vi "Votlage - Pressure Amb Conversion.vi"(11 "mean":dbl) -> (3 "Numeric":dbl)   [LabVIEW 2018]
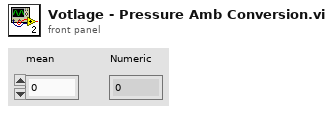
[diagram p1: front panel]
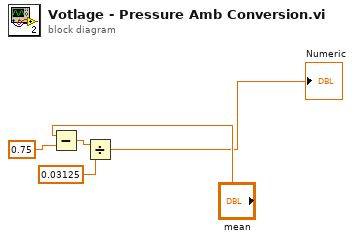
[diagram p0: block diagram]
diagram:
  n1 = Subtract(x="mean", y=0.75 ("minimum value")) -> (x-y=w2:dbl)
  n2 = Divide(x=w2, y=0.03125 ("minimum value")) -> (x/y=→"Numeric":dbl)
